vi "EletoMatr_n channel.vi"(0 "Input Array X":dbl[][](array[numeric]), 5 "Input data":dbl[](array[numeric]), 7 "No. channels":i32=1, 9 "In Row":i32, 11 "In Column":i32, 12 "Input Direction":bool=TRUE) -> (3 "Completed":bool=TRUE, 4 "Out Array X":dbl[][](array[numeric]), 10 "Out Row":i32, 14 "Output Direction":bool=TRUE, 15 "Out Column":i32)   [LabVIEW 2018]
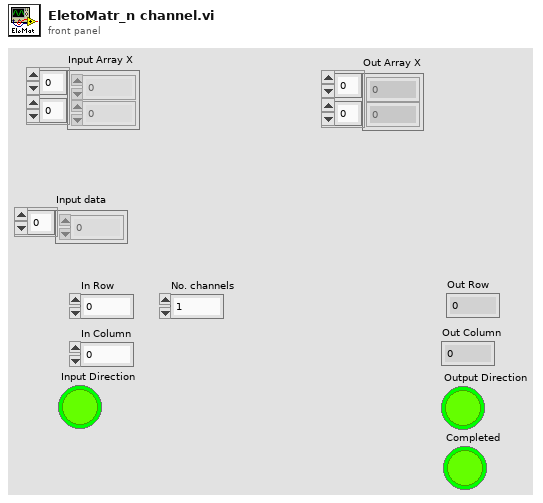
[diagram p1: front panel]
types:
  T1 = typedef "NI_Matrix.lvlib/RealMatrix.ctl" = dbl[][]
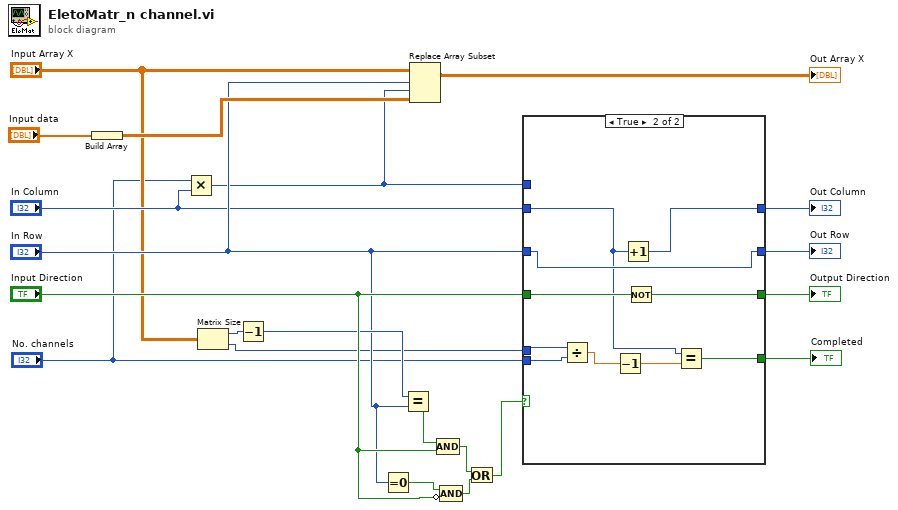
[diagram p0: block diagram]
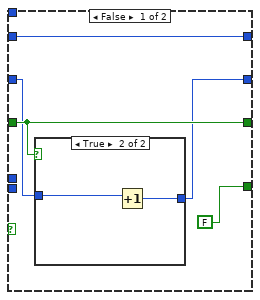
[diagram p2: hidden frame]
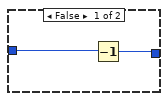
[diagram p3: hidden frame]
diagram:
  n1 = Build Array("Input data") -> (w9:dbl[][])
  n2 = Multiply(x="No. channels", y="In Column") -> (x*y=w5:i32)
  n3 = Matrix Size(0:"Input Array X") -> (1:w15:i32, 2:w3:i32)
  n4 = Decrement(x=w15) -> (x-1=w10:i32)
  n5 = Equal To 0?(x="In Row") -> (x = 0?=w11:bool)
  n6 = Equal?(x=w10, y="In Row") -> (x = y?=w14:bool)
  n7 = Replace Array Subset(array="Input Array X", new element=w9, index (row)="In Row", index (col)=w5) -> (→"Out Array X":T1)
  n8 = Compound Arithmetic op=AND(w14, "Input Direction") -> (w12:bool)
  n9 = Compound Arithmetic op=AND(w11, invert "Input Direction") -> (w17:bool)
  n10 = Or(x=w12, y=w17) -> (x .or. y?=w16:bool)
  n11 = case shown="True" w16 {
    tunnel: "Input Direction" -> [w26 w40]
    tunnel: "In Row" -> [w24 w36]
    tunnel: [w22 w37] -> w21
    tunnel: "In Column" -> [w22 w31]
    tunnel: [w26 w39] -> w20
    tunnel: [w23 w36] -> w19
    tunnel: w3 -> [_ w35]
    tunnel: [FALSE w38] -> w18
    tunnel: w5 -> [_ _]
    tunnel: "No. channels" -> [_ w34]
    frame False {
      n12 = case shown="True" w26 {
        tunnel: [w28 w30] -> w23
        tunnel: w24 -> [w27 w29]
        frame False {
          n13 = Decrement(x=w27) -> (x-1=w28:i32)
        }
        frame True {
          n14 = Increment(x=w29) -> (x+1=w30:i32)
        }
      }
    }
    frame True {
      n15 = Divide(x=w35, y=w34) -> (x/y=w33:dbl)
      n16 = Decrement(x=w33) -> (x-1=w32:dbl)
      n17 = Increment(x=w31) -> (x+1=w37:i32)
      n18 = Not(x=w40) -> (.not. x?=w39:bool)
      n19 = Equal?(x=w31, y=w32) -> (x = y?=w38:bool)
    }
  }
  "Out Row" <- w19
  "Out Column" <- w21
  "Output Direction" <- w20
  "Completed" <- w18
